vi "lamp.vi"(4 "lamp":T1, 5 "GPIB in":string="18") -> (0 "lamp okay":bool, 2 "GPIB out":string="18")   [LabVIEW 2015]
uses:
  lamp2.ctl
panel:
  out "Checking Lamp":dbl(slide) scale=0.0..60.0
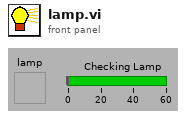
[diagram p1: front panel]
types:
  T1 = typedef "lamp2.ctl" = bool
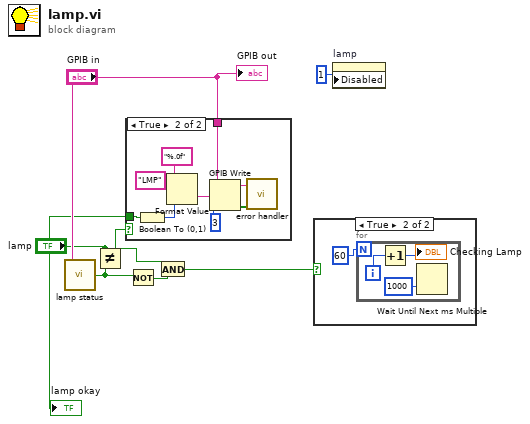
[diagram p0: block diagram]
diagram:
  n1 = call "lamp status.vi"("GPIB in"="GPIB in") -> ("lamp"=w3:T1)  [unwired: 2 in, 2 out]
  n2 = Not Equal?(x="lamp", y=w3) -> (x != y?=w2:T1)
  n3 = case shown="True" w2 {
    tunnel: "lamp" -> [_ w15]
    tunnel: "GPIB in" -> [_ w12]
    frame False {
    }
    frame True {
      n4 = Boolean To (0,1)(Boolean=w15) -> (0, 1=w11:i16)
      n5 = Format Value(string ("")="LMP", format string="%.0f", value (0)=w11) -> (output string=w13:string)
      n6 = GPIB Write(0:w12, 1:w13, 2:3) -> (5:w14:bool[])  [unwired: 2 in, 1 out]
      n7 = call "error handler.vi"("status array"=w14, "GPIB in"=w12) -> ()  [unwired: 3 in, 3 out]
    }
  }
  n8 = Not(x=w3) -> (.not. x?=w5:T1)
  n9 = And(x="lamp", y=w5) -> (x .and. y?=w4:T1)
  n10 = case shown="True" w4 {
    frame False {
    }
    frame True {
      n11 = for {
        N: 60 -> [_]
        i -> [w18]
        n12 = Increment(x=w18) -> (x+1=→"Checking Lamp":i32)
        n13 = Wait Until Next ms Multiple(millisecond multiple=1000) -> ()  [unwired: 1 out]
      }
    }
  }
  n14 = property on="lamp" class="Bool (strict)"("Disabled"=1) -> ()  [unwired: 2 in, 2 out]
  "GPIB out" <- "GPIB in"
  "lamp okay" <- "lamp"
